vi "AB_User_Log_Open.vi"(8 "error in (no error)":errorcluster, 9 "build spec name":string, 10 "Object":T1, 11 "file":path) -> (0 "error out":errorcluster)   [LabVIEW 2020]
uses:
  <resource>/Framework/Providers/API/ItemRef.ctl
  <vilib>/AppBuilder/logging/AB_Log_File_Action.ctl
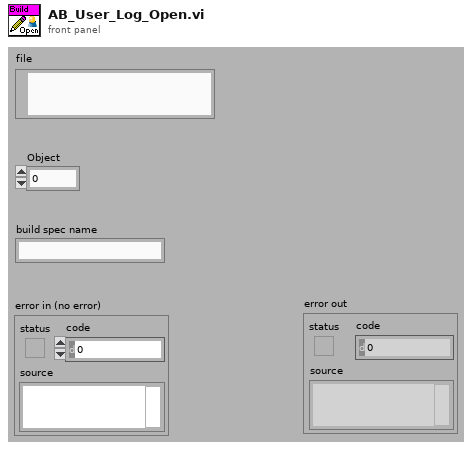
[diagram p1: front panel]
types:
  T1 = typedef "ItemRef.ctl" = u64
  T2 = typedef "AB_Log_File_Action.ctl" = enum16{"write", "open", "close"}
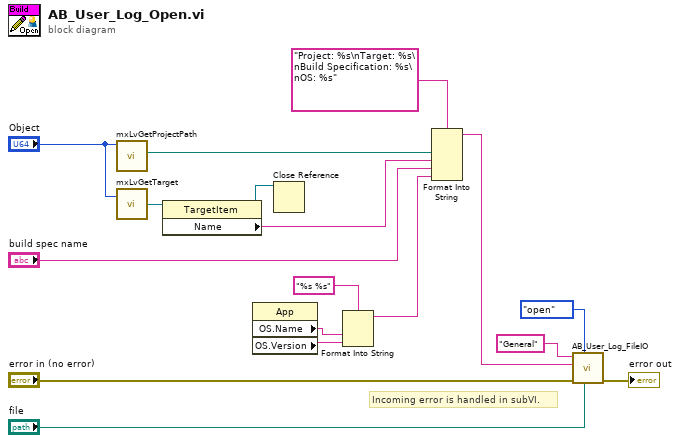
[diagram p0: block diagram]
diagram:
  # "Incoming error is handled in subVI."
  n1 = call <resource>:"mxLvGetProjectPath.vi"("Item"="Object") -> ("Project Path"=w7:path)  [unwired: 1 in, 9 out]
  n2 = call <resource>:"mxLvGetTarget.vi"("Item"="Object") -> ("Target"=w16:refnum<vi>)  [unwired: 1 in, 2 out]
  n3 = property class="TargetItem"(reference=w16) -> (reference out=w14:refnum<vi>, "Name"=w15:string)  [unwired: 1 in, 1 out]
  n4 = property class="App"() -> ("OS.Name"=w6:string, "OS.Version"=w5:string)  [unwired: 2 in, 2 out]
  n5 = Close Reference(reference=w14) -> ()  [unwired: 1 in, 1 out]
  n6 = Format Into String(format string="%s %s", w6, w5) -> (resulting string=w3:string)  [unwired: 2 in, 1 out]
  n7 = Format Into String(format string="Project: %s\nTarget: %s\nBuild Specification: %s\nOS: %s", w7, w15, "build spec name", w3) -> (resulting string=w10:string)  [unwired: 2 in, 1 out]
  n8 = call <vilib>:"AB_User_Log_FileIO.vi"("file"="file", "fileAction"=AB_Log_File_Action."open", "error in (no error)"="error in (no error)", "data"=w10, "newSection"="General" ("data")) -> ("error out"=→"error out":errorcluster)  [unwired: 6 out]
